vi "MT Format Eye Diagram (WDT).vi"(0 "waveform":waveform(dbl)={"t0"=timestamp(0 s since 1904-01-01), "dt"=0.0, "Y"=[]}, 1 "eye diagram reference":refnum<vi>, 5 "symbol rate (Hz)":dbl=1.0 format="%.2f", 7 "eye length":i32=1, 11 "error in (no error)":errorcluster, 12 "autoscale":bool) -> (4 "eye diagram":cluster{"t0":dbl, "dt":dbl, "Y":dbl[]}[](array[cluster]) {"Y" format="%.2f"; "dt" format="%.2f"; "t0" format="%.2f"}, 15 "error out":errorcluster)   [LabVIEW 2020, in "niDMT.lvlib"]
doc: "Specifies a real-valued waveform, divides it into segments, and displays those segments as plots on a waveform graph. This VI determines the segment length based on the <B>symbol rate</B> and <B>eye length</B> parameters."
uses:
  <vilib>/addons/Modulation/niDMT.lvlib
  <vilib>/addons/Modulation/Digital/General/subVIs/mod_Segment Array(WDT).vi
  <vilib>/addons/Modulation/niAMT.lvlib
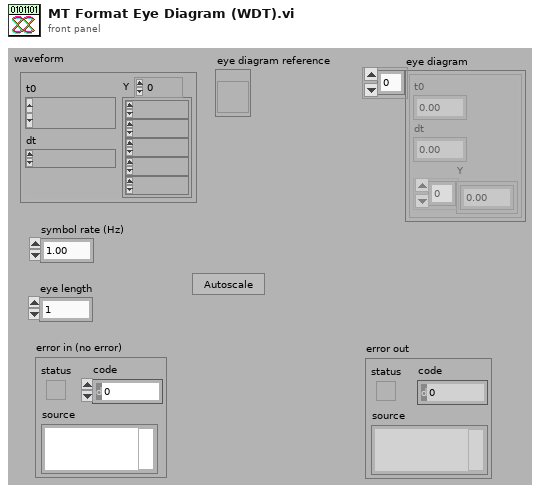
[diagram p1: front panel]
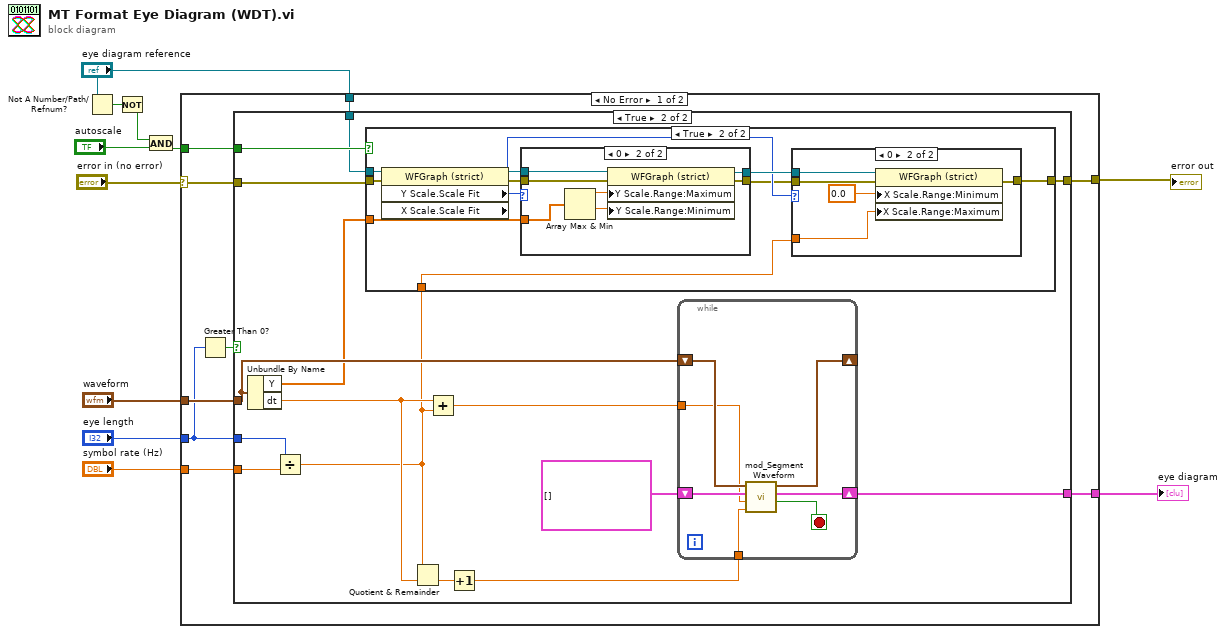
[diagram p0: block diagram]
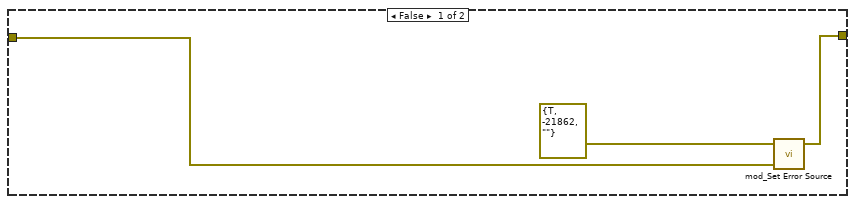
[diagram p2: hidden frame]
diagram:
  n1 = Not A Number/Path/Refnum?(number/path/refnum="eye diagram reference") -> (NaN/Path/Refnum?=w4:bool)
  n2 = Not(x=w4) -> (.not. x?=w3:bool)
  n3 = And(x=w3, y="autoscale") -> (x .and. y?=w1:bool)
  n4 = case shown="No Error" "error in (no error)" {
    selector: "error in (no error)" -> [w17 w73]
    tunnel: "eye length" -> [w13 _]
    tunnel: "symbol rate (Hz)" -> [w20 _]
    tunnel: "waveform" -> [w19 _]
    tunnel: [w18 _] -> w8
    tunnel: [w12 w73] -> w6
    tunnel: "eye diagram reference" -> [w16 _]
    tunnel: w1 -> [w15 _]
    frame No Error {
      n5 = Greater Than 0?(x=w13) -> (x > 0?=w14:bool)
      n6 = case shown="True" w14 {
        tunnel: w13 -> [_ w37]
        tunnel: w20 -> [_ w36]
        tunnel: w19 -> [_ w34]
        tunnel: [_ w32] -> w18
        tunnel: w17 -> [w21 w28]
        tunnel: [w22 w25] -> w12
        tunnel: w16 -> [_ w26]
        tunnel: w15 -> [_ w27]
        frame False {
          n7 = call <vilib>:"mod_Set Error Source.vi"("initial error in (no error)"=w21, "final error in (no error)"=errorcluster {"status"=TRUE, "code"=-21862, "source"=""}) -> ("error out"=w22:errorcluster)  [unwired: 3 out]
        }
        frame True {
          n8 = Unbundle By Name(w34) -> ("Y"=w24:dbl[], "dt"=w30:dbl)
          n9 = Divide(x=w37, y=w36) -> (x/y=w29:dbl)
          n10 = case shown="True" w27 {
            tunnel: [w39 w40] -> w25
            tunnel: w26 -> [_ w49]
            tunnel: w28 -> [w39 w48]
            tunnel: w24 -> [_ w50]
            tunnel: w29 -> [_ w42]
            frame False {
            }
            frame True {
              n11 = property class="WFGraph (strict)"(reference=w49, error in=w48) -> (reference out=w47:refnum<vi>, error out=w46:errorcluster, "Y Scale.Scale Fit"=w45:u8, "X Scale.Scale Fit"=w43:u8)
              n12 = case shown="0" w45 {
                tunnel: [w58 w65] -> w41
                tunnel: w50 -> [_ w64]
                tunnel: w47 -> [w57 w63]
                tunnel: w46 -> [w58 w62]
                tunnel: [w57 w61] -> w44
                frame 1, Default {
                }
                frame 0 {
                  n13 = Array Max & Min(array=w64) -> (max value=w60:dbl, min value=w59:dbl)  [unwired: 2 out]
                  n14 = property class="WFGraph (strict)"(reference=w63, error in=w62, "Y Scale.Range:Maximum"=w60, "Y Scale.Range:Minimum"=w59) -> (reference out=w61:refnum<vi>, error out=w65:errorcluster)
                }
              }
              n15 = case shown="0" w43 {
                tunnel: [w51 w52] -> w40
                tunnel: w42 -> [_ w55]
                tunnel: w44 -> [_ w54]
                tunnel: w41 -> [w51 w53]
                frame 1, Default {
                }
                frame 0 {
                  n16 = property class="WFGraph (strict)"(reference=w54, error in=w53, "X Scale.Range:Minimum"=0.0, "X Scale.Range:Maximum"=w55) -> (error out=w52:errorcluster)  [unwired: 1 out]
                }
              }
            }
          }
          n17 = Quotient & Remainder(x=w29, y=w30) -> (floor(x/y)=w35:dbl)  [unwired: 1 out]
          n18 = Add(x=w30, y=w29) -> (x+y=w38:dbl)
          n19 = Increment(x=w35) -> (x+1=w31:dbl)
          n20 = while {
            tunnel: w38 -> [w69]
            tunnel: w31 -> [w68]
            shift-right: [w71] -> _
            shift-left: w34 -> [w72]
            shift-right: [w66] -> w32
            shift-left: cluster{"t0":dbl, "dt":dbl, "Y":dbl[]}[] [] ("empty graphs in") -> [w70]
            stop <- w67 stop-if-true
            n21 = call-poly <vilib>:"mod_Segment Waveform.vi"("min samples per segment"=w68, "segment time"=w69, "graphs in"=w70, "waveform"=w72) -> ("done?"=w67:bool, "graphs out"=w66:cluster{"t0":dbl, "dt":dbl, "Y":dbl[]}[], "waveform out"=w71:waveform(dbl))  [unwired: 5 out]
          }
        }
      }
    }
    frame Error {
    }
  }
  "eye diagram" <- w8
  "error out" <- w6
